vi "Shift distance data insert.vi"(8 "error in (no error)":errorcluster, 11 "移位距离":dbl) -> (0 "error out":errorcluster)   [LabVIEW 2016, in "AIRMAR WeatherCaster.lvlib"]
uses:
  AIRMAR WeatherCaster.lvlib
panel:
  in  "data in":cluster{"时间":timestamp, "移位距离":dbl}
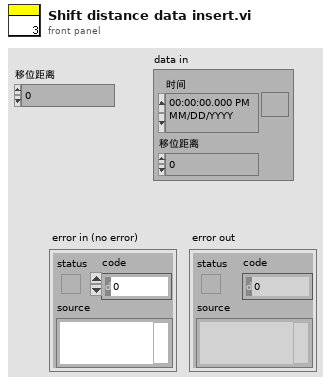
[diagram p1: front panel]
types:
  T1 = typedef "数据库类型.ctl" = enum16{"Access", "SQLite"}
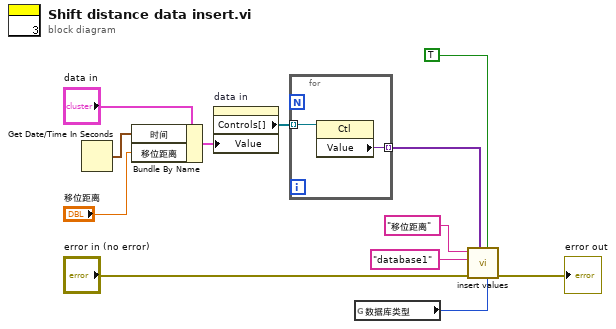
[diagram p0: block diagram]
diagram:
  n1 = Get Date/Time In Seconds() -> (seconds since 1Jan1904=w10:timestamp)
  n2 = Bundle By Name(cluster="data in", "时间"=w10, "移位距离"="移位距离") -> (w9:cluster{"时间":timestamp, "移位距离":dbl})
  n3 = property on="data in" class="Clust (严格)"("Value"=w9) -> ("Controls[]"=w12:refnum<vi>[])  [unwired: 2 in, 2 out]
  n4 = for {
    tunnel: w12 -> [w14] mode=indexing
    tunnel: [w13] -> w7 mode=indexing
    n5 = property class="Ctl"(reference=w14) -> ("Value"=w13:variant)  [unwired: 1 in, 2 out]
  }
  n6 = global read "气象全局变量.vi" "数据库类型"() -> (w1:T1)
  n7 = call "insert values.vi"("数据库类型"=w1, "是否创建唯一键"=TRUE, "data"=w7, "错误输入（无错误）"="error in (no error)", "database"="database1", "Tabe Name"="移位距离" ("table")) -> ("错误输出"=→"error out":errorcluster)  [unwired: 5 in]
